vi "4072_Config.vi"(8 "error in (no error)":errorcluster, 11 "Device Ref out":T2 format="%.0x") -> (0 "error out":errorcluster, 2 "Instrument Handle Out":T1)   [LabVIEW 2015, in "NI PXI-4072 DMM Custom Device.lvlib"]
uses:
  NI PXI-4072 DMM Custom Device.lvlib
  <vilib>/NI Veristand/Custom Device API/Custom Device Item Ref.ctl
  <instrlib>/niDMM/nidmm.llb/niDMM Resolution in Digits.ctl
  4072_Global.vi
  <vilib>/NI Veristand/Custom Device API/Get Item Property (String).vi
  <vilib>/NI Veristand/Custom Device API/Get Item Property (U16).vi
  <vilib>/NI Veristand/Custom Device API/Get Item Property (Double).vi
  <instrlib>/niDMM/nidmm.llb/niDMM Configure Measurement Digits.vi
  <vilib>/NI Veristand/Custom Device API/Custom Device API.lvlib
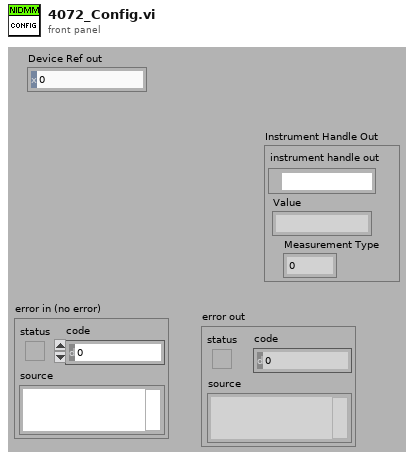
[diagram p1: front panel]
types:
  T1 = cluster{"instrument handle out":refnum<k15>, "Value":string, "Measurement Type":u16}
  T2 = typedef "Custom Device API.lvlib/Custom Device Item Ref.ctl" = u64
  T3 = enum16{"3 1/2", "4 1/2", "5 1/2", "6 1/2", "7 1/7"}
  T4 = typedef "niDMM Resolution in Digits.ctl" = dbl
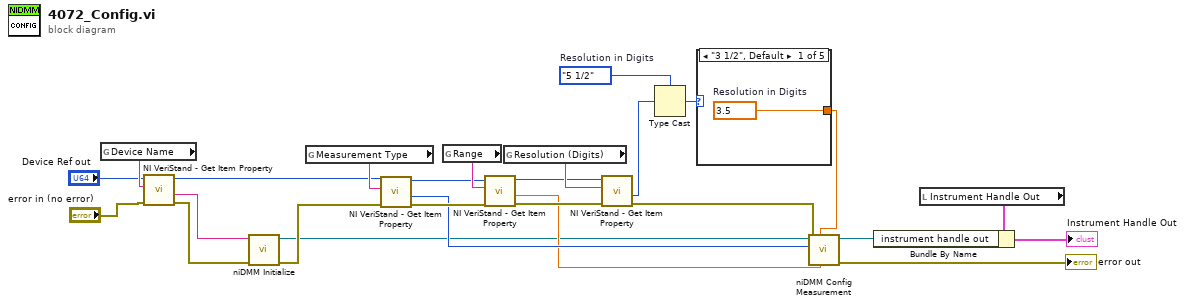
[diagram p0: block diagram]
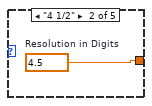
[diagram p2: hidden frame]
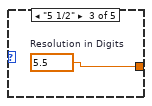
[diagram p3: hidden frame]
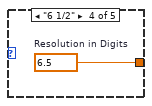
[diagram p4: hidden frame]
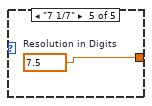
[diagram p5: hidden frame]
diagram:
  w3 = T3."5 1/2"  # Resolution in Digits
  n1 = global read "4072_Global.vi" "Device Name"() -> (w26:string)
  n2 = call-poly <vilib>:"NI VeriStand - Get Item Property.vi"("error in (no error)"="error in (no error)", "Property Name"=w26, "Item Ref in"="Device Ref out") -> ("error out"=w23:errorcluster, "Value"=w21:string, "Item Ref out"=w5:T2)  [unwired: 5 in, 1 out]
  n3 = call <instrlib>:"niDMM Initialize.vi"("error in (no error)"=w23, "Instrument Descriptor"=w21) -> ("error out"=w22:errorcluster, "instrument handle out"=w10:refnum<k15>)  [unwired: 8 in]
  n4 = global read "4072_Global.vi" "Measurement Type"() -> (w19:string)
  n5 = call-poly <vilib>:"NI VeriStand - Get Item Property.vi"("error in (no error)"=w22, "Property Name"=w19, "Item Ref in"=w5) -> ("error out"=w17:errorcluster, "Value"=w12:u16, "Item Ref out"=w18:T2)  [unwired: 5 in, 1 out]
  n6 = global read "4072_Global.vi" "Range"() -> (w20:string)
  n7 = call-poly <vilib>:"NI VeriStand - Get Item Property.vi"("error in (no error)"=w17, "Property Name"=w20, "Item Ref in"=w18) -> ("error out"=w14:errorcluster, "Value"=w11:dbl, "Item Ref out"=w15:T2)  [unwired: 5 in, 1 out]
  n8 = global read "4072_Global.vi" "Resolution (Digits)"() -> (w16:string)
  n9 = call-poly <vilib>:"NI VeriStand - Get Item Property.vi"("error in (no error)"=w14, "Property Name"=w16, "Item Ref in"=w15) -> ("error out"=w13:errorcluster, "Value"=w4:u16)  [unwired: 5 in, 2 out]
  n10 = Type Cast(type=w3, x=w4) -> (*(type *) &x=w2:T3)
  n11 = case shown="\"3 1/2\", Default" w2 {
    tunnel: [w27 w28 w29 w30 w31] -> w1
    frame "3 1/2", Default {
      w27 = T4 3.5 items=["3 1/2"=3.5, "4 1/2"=4.5, "5 1/2"=5.5, "6 1/2"=6.5, "7 1/2"=7.5]  # Resolution in Digits
    }
    frame "4 1/2" {
      w28 = T4 4.5 items=["3 1/2"=3.5, "4 1/2"=4.5, "5 1/2"=5.5, "6 1/2"=6.5, "7 1/2"=7.5]  # Resolution in Digits
    }
    frame "5 1/2" {
      w29 = T4 5.5 items=["3 1/2"=3.5, "4 1/2"=4.5, "5 1/2"=5.5, "6 1/2"=6.5, "7 1/2"=7.5]  # Resolution in Digits
    }
    frame "6 1/2" {
      w30 = T4 6.5 items=["3 1/2"=3.5, "4 1/2"=4.5, "5 1/2"=5.5, "6 1/2"=6.5, "7 1/2"=7.5]  # Resolution in Digits
    }
    frame "7 1/7" {
      w31 = T4 7.5 items=["3 1/2"=3.5, "4 1/2"=4.5, "5 1/2"=5.5, "6 1/2"=6.5, "7 1/2"=7.5]  # Resolution in Digits
    }
  }
  n12 = call-poly <instrlib>:"niDMM Config Measurement.vi"("Range"=w11, "Resolution in Digits"=w1, "error in (no error)"=w13, "Function"=w12, "instrument handle"=w10) -> ("error out"=→"error out":errorcluster, "instrument handle out"=w7:refnum<k15>)  [unwired: 5 in]
  n13 = local read "Instrument Handle Out"() -> (w9:T1)
  n14 = Bundle By Name(cluster=w9, "instrument handle out"=w7) -> (→"Instrument Handle Out":T1)
